vi "Temperature_main.vi"(0 "VISA resource name":refnum<visa-resource-name>="COM1") -> ()   [LabVIEW 2012]
doc: "The Basic Serial Read and Write example performs a Serial Port Read, a Serial Port Write, or a combination of these actions. The user selects the actions (read or write) on the front panel. If both are selected, the VI will write the data first, read data, and then close the VISA session that is opened to the port. This VI will wait until the specified number of bytes is received at the port. Only the number of bytes specified will be read.\n\nINSTRUCTIONS:\n1) Select the serial resource and configuration parameters (baud rate, data bits, parity, stop bits, flow control).\n2) Select the operations to be performed. \n3) Connect the serial port to your device. If no device is available, perform a loopback test by doing one of the following. Short pins 2 and 3 on a RS-232 cable or short pin 4 to pin 8 and pin 5 to pin 9 on a RS-485/422 cable. \n4) Run the VI to see the data read. (The \"read string\" will match the \"string to write\" if a loopback test was performed.)\n\nNote: The parameters set for the serial port must match the parameters of the connected instrument or device. In this example, the bytes to read parameter specifies the number of bytes that the serial port reads. If there were more bytes at the port than the number specified in bytes to read, those bytes would not be read. Also, if you specify to read more bytes than the number of bytes actually read, you might receive a timeout error message.\n\nOn the block diagram, the Configure Serial Port VI sets the configuration parameters. The front panel displays the controls used to configure the basic parameters, such as baud rate, data bits, and parity. Constants configure the other parameters the user probably does not need set. After the VISA Configure Serial Port VI opens the VISA session and configures the port, the VI passes the VISA resource name to other VIs that perform operations on that VISA resource. The VISA Write function sends a command to the serial device and the VISA Read function returns data based on the command. The VISA Close function then closes the reference to the serial device. It is important to close the reference; otherwise communication through with that port through protocols other than VISA might not be possible."
uses:
  <vilib>/Instr/_visa.llb/VISA Configure Serial Port (Instr).vi
panel:
  out "T4, C":string
  out "T3, C":string
  out "T2, C":string
  out "T1, C":string
  out "Измеритель температуры\nCenter 304 (309)":bool
  out "T4":bool
  out "T3":bool
  out "T2":bool
  out "T1":bool
  out "Boolean array for 2nd byte":bool[](array[boolean])
  out "Boolean array for 1st byte":bool[](array[boolean])
  out "unsigned byte array":u8[](array[numeric])
  # "Select the serial resource and the operations (Read, Write, or both) to be performed.  If both are selected, the VI will write the data first, read data and then close the VISA session that is opened to the port.  This VI will wait until the specified number of bytes is received at the port. Only the number of bytes specified will be read."
  # "For additional information select File >> VI Properties >> Documentation"
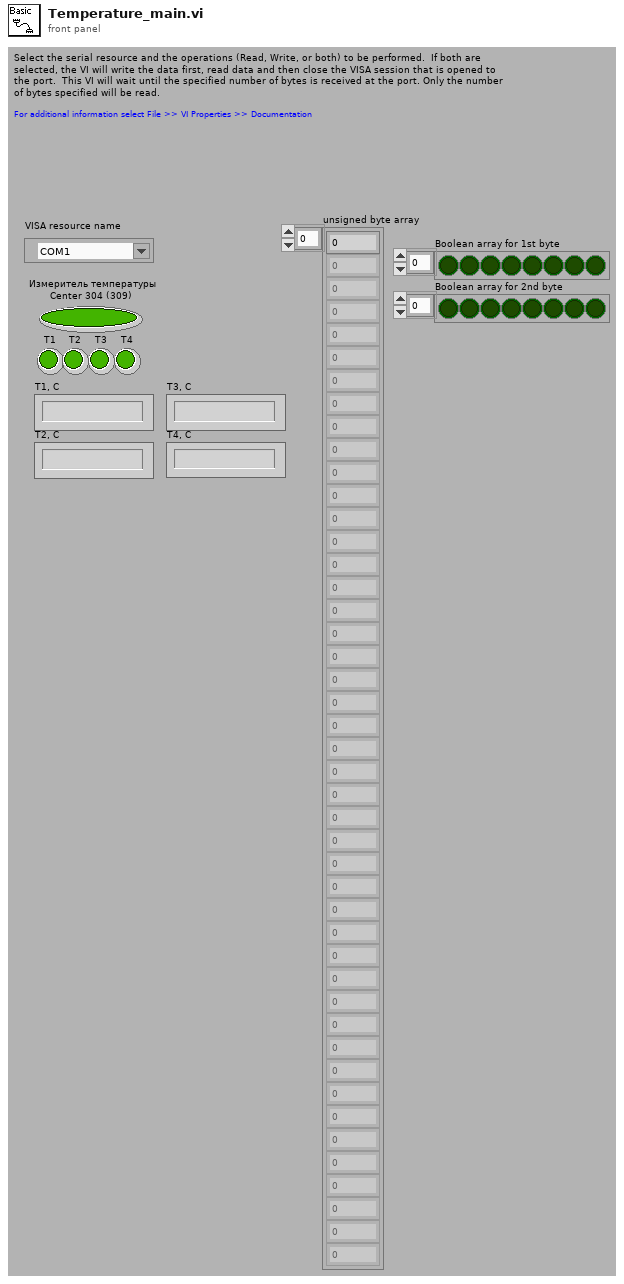
[diagram p1: front panel]
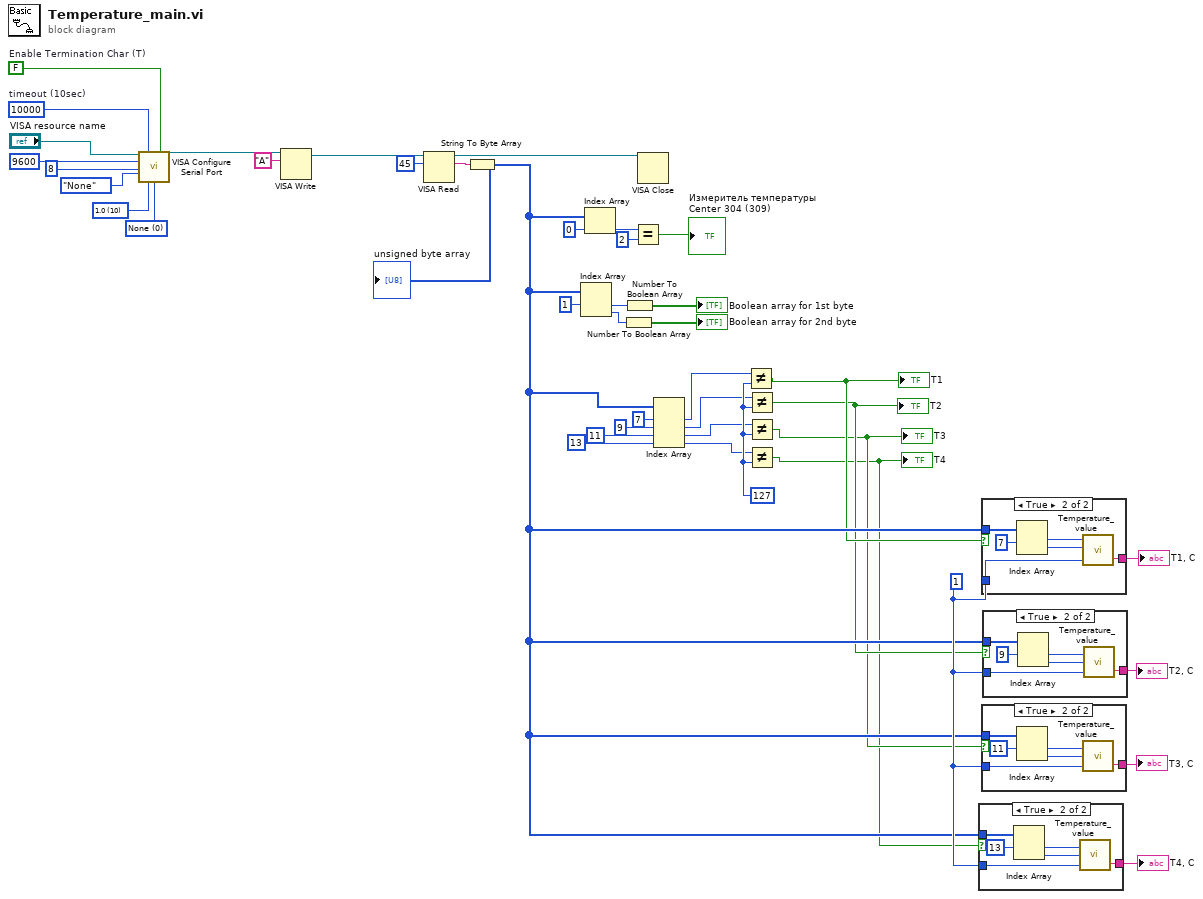
[diagram p0: block diagram]
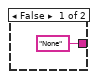
[diagram p2: hidden frame]
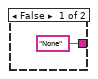
[diagram p3: hidden frame]
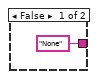
[diagram p4: hidden frame]
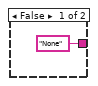
[diagram p5: hidden frame]
diagram:
  w12 = u8 127 ("y")
  w18 = i16 1 ("precision")
  w27 = u16 0 items=["None", "XON/XOFF", "RTS/CTS", "XON/XOFF & RTS/CTS", "DTR/DSR", "XON/XOFF & DTR/DSR"] ("flow control (0:none)")
  w28 = u16 10 items=["1.0"=10, "1.5"=15, "2.0"=20] ("stop bits (10: 1 bit)")
  w38 = FALSE  # Enable Termination Char (T)
  w39 = u32 10000  # timeout (10sec)
  n1 = call-poly "VISA Configure Serial Port"("VISA resource name"="VISA resource name", "timeout (10sec)"=w39, "Enable Termination\nChar (T)"=w38, "baud rate (9600)"=u32 9600, "data bits (8)"=u16 8, "parity (0:none)"=enum16{"None", "Odd", "Even", "Mark", "Space"}."None", "stop bits (10: 1 bit)"=w28, "flow control (0:none)"=w27) -> ("VISA resource name out"=w41:refnum<visa-resource-name>)  [unwired: 6 in, 1 out]
  n2 = VISA Write(VISA resource name=w41, write buffer="A") -> (VISA resource name out=w37:refnum<visa-resource-name>)  [unwired: 1 in, 2 out]
  n3 = VISA Read(VISA resource name=w37, byte count=u32 45) -> (VISA resource name out=w40:refnum<visa-resource-name>, read buffer=w36:string)  [unwired: 1 in, 2 out]
  n4 = String To Byte Array(string=w36) -> (unsigned byte array=w10:u8[])
  "unsigned byte array" <- w10
  n5 = Index Array(array=w10, index #1=1 ("index")) -> (element #1=w34:u8, element #2=w21:u8)  [unwired: 1 in]
  n6 = Index Array(array=w10, index=0) -> (element=w24:u8)
  n7 = Number To Boolean Array(number=w21) -> (Boolean array=→"Boolean array for 2nd byte":bool[])
  n8 = Number To Boolean Array(number=w34) -> (Boolean array=→"Boolean array for 1st byte":bool[])
  n9 = Equal?(x=w24, y=u8 2) -> (x = y?=→"Измеритель температуры\nCenter 304 (309)":bool)
  n10 = VISA Close(VISA resource name=w40) -> ()  [unwired: 1 in, 1 out]
  n11 = Index Array(array=w10, index #1=7 ("index"), index #2=9 ("index"), index #3=11 ("index"), index #4=13 ("index")) -> (element #1=w11:u8, element #2=w8:u8, element #3=w7:u8, element #4=w6:u8)
  n12 = Not Equal?(x=w11, y=w12) -> (x != y?=w5:bool)
  "T1" <- w5
  n13 = Not Equal?(x=w8, y=w12) -> (x != y?=w4:bool)
  "T2" <- w4
  n14 = Not Equal?(x=w7, y=w12) -> (x != y?=w3:bool)
  "T3" <- w3
  n15 = Not Equal?(x=w6, y=w12) -> (x != y?=w2:bool)
  "T4" <- w2
  n16 = case shown="True" w2 {
    tunnel: ["None" ("Temperature string") w48] -> w16
    tunnel: w10 -> [_ w47]
    tunnel: w18 -> [_ w44]
    frame False {
    }
    frame True {
      n17 = Index Array(array=w47, index #1=13 ("index")) -> (element #1=w46:u8, element #2=w45:u8)  [unwired: 1 in]
      n18 = call "Temperature_value.vi"("precision"=w44, "2nd byte"=w45, "1st byte"=w46) -> ("Temperature string"=w48:string)  [unwired: 1 out]
    }
  }
  "T4, C" <- w16
  n19 = case shown="True" w5 {
    tunnel: w10 -> [_ w56]
    tunnel: ["None" ("Temperature string") w52] -> w20
    tunnel: w18 -> [_ w51]
    frame False {
    }
    frame True {
      n20 = Index Array(array=w56, index #1=7 ("index")) -> (element #1=w54:u8, element #2=w53:u8)  [unwired: 1 in]
      n21 = call "Temperature_value.vi"("precision"=w51, "2nd byte"=w53, "1st byte"=w54) -> ("Temperature string"=w52:string)  [unwired: 1 out]
    }
  }
  "T1, C" <- w20
  n22 = case shown="True" w3 {
    tunnel: ["None" ("Temperature string") w62] -> w17
    tunnel: w10 -> [_ w61]
    tunnel: w18 -> [_ w58]
    frame False {
    }
    frame True {
      n23 = Index Array(array=w61, index #1=11 ("index")) -> (element #1=w60:u8, element #2=w59:u8)  [unwired: 1 in]
      n24 = call "Temperature_value.vi"("precision"=w58, "2nd byte"=w59, "1st byte"=w60) -> ("Temperature string"=w62:string)  [unwired: 1 out]
    }
  }
  "T3, C" <- w17
  n25 = case shown="True" w4 {
    tunnel: ["None" ("Temperature string") w69] -> w19
    tunnel: w10 -> [_ w68]
    tunnel: w18 -> [_ w65]
    frame False {
    }
    frame True {
      n26 = Index Array(array=w68, index #1=9 ("index")) -> (element #1=w67:u8, element #2=w66:u8)  [unwired: 1 in]
      n27 = call "Temperature_value.vi"("precision"=w65, "2nd byte"=w66, "1st byte"=w67) -> ("Temperature string"=w69:string)  [unwired: 1 out]
    }
  }
  "T2, C" <- w19
